vi "Test Cross Correlation.vi"() -> ()   [LabVIEW 2019]
uses:
  src/xy_utilities.lvlib
  src/subVIs/Difference Quotient (multiple).vi
  src/subVIs/Subtract float (single).vi
panel:
  out "R_AB":cluster{"X-array":dbl[], "Y-array":dbl[]}(graph)
  in  "index":i32
  out "XY Graph 2":cluster{dbl[], dbl[]}[](graph)
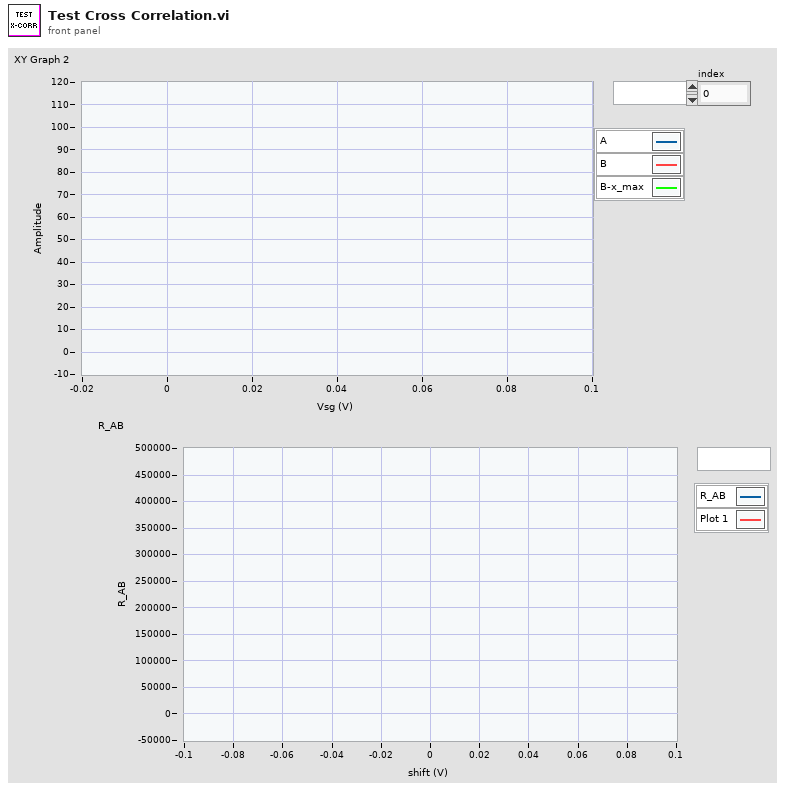
[diagram p1: front panel]
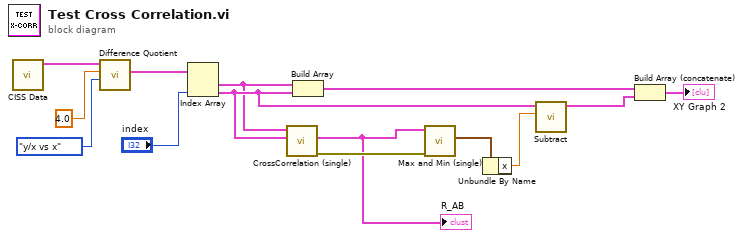
[diagram p0: block diagram]
diagram:
  n1 = call "CISS Data.vi"() -> ("G vs X"=w13:cluster{dbl[], dbl[]}[])  [unwired: 10 in, 1 out]
  n2 = call-poly "Difference Quotient.vi"("Type"=enum16{"y/x vs x", "x/y vs y"}."y/x vs x", "Window [h] (2)"=4.0, "XY-data"=w13) -> ("Difference Quotient"=w10:cluster{"X-array":dbl[], "Y-array":dbl[]}[])  [unwired: 6 in, 2 out]
  n3 = Index Array(array=w10, index #2="index") -> (element #1=w4:cluster{"X-array":dbl[], "Y-array":dbl[]}, element #2=w6:cluster{"X-array":dbl[], "Y-array":dbl[]})  [unwired: 1 in]
  n4 = call "CrossCorrelation (single).vi"("XY-data b"=w6, "XY-data a"=w4) -> ("error out"=w5:errorcluster, "R_ab"=w2:cluster{"X-array":dbl[], "Y-array":dbl[]})  [unwired: 7 in, 1 out]
  "R_AB" <- w2
  n5 = Build Array(w4, w6) -> (w1:cluster{"X-array":dbl[], "Y-array":dbl[]}[])
  n6 = call "Max and Min (single).vi"("error in (no error)"=w5, "XY-data"=w2) -> ("y_max (x,y)"=w9:cluster{"x":dbl, "y":dbl})  [unwired: 6 in, 3 out]
  n7 = Unbundle By Name(w9) -> ("x"=w8:dbl)
  n8 = call-poly "Subtract.vi"("x (0)"=w8, "XY-data"=w6) -> ("XY-data out"=w3:cluster{"X-array":dbl[], "Y-array":dbl[]})  [unwired: 8 in, 1 out]
  n9 = Build Array (concatenate)(w1, w3) -> (→"XY Graph 2":cluster{"X-array":dbl[], "Y-array":dbl[]}[])
